vi "Main.vi"() -> ()   [LabVIEW 2020]
uses:
  Library Builder/Library Builder.lvclass
  Package Builder/Package Builder.lvclass
panel:
  in  "Stop":bool
  out "Time Elapsed":dbl format="%<%H:%M:%S>t"
  out "Status":string
  out "error out":errorcluster
  in  "Package Description":string="The NI-XNET Monitor Custom Device allows a user to run subordinate XNET session for each port in the system to be able to monitor port status, error counters, frame counter and other interface health indicators. This custom device also allows estimating the bus load present for the CAN buses added to the system. It's implemented as HW Inline Asynchronous Custom Device."
  in  "Build Config":T1(array[cluster])=[{"Version"=2020, "TCP/IP Port"=3363, "BuildPkg"=TRUE}, {"Version"=2021, "TCP/IP Port"=3364, "BuildPkg"=TRUE}, {"Version"=2023, "TCP/IP Port"=3365, "BuildPkg"=TRUE}]
  in  "Output Directory":path=path "\\\\vmware-host\\Shared Folders/_Repo/NI-XNET-Monitor-Custom-Device/Release"
  in  "Project Path":path=path "\\\\vmware-host\\Shared Folders/_Repo/NI-XNET-Monitor-Custom-Device/Source/NI-XNET Monitor Custom Device.lvproj"
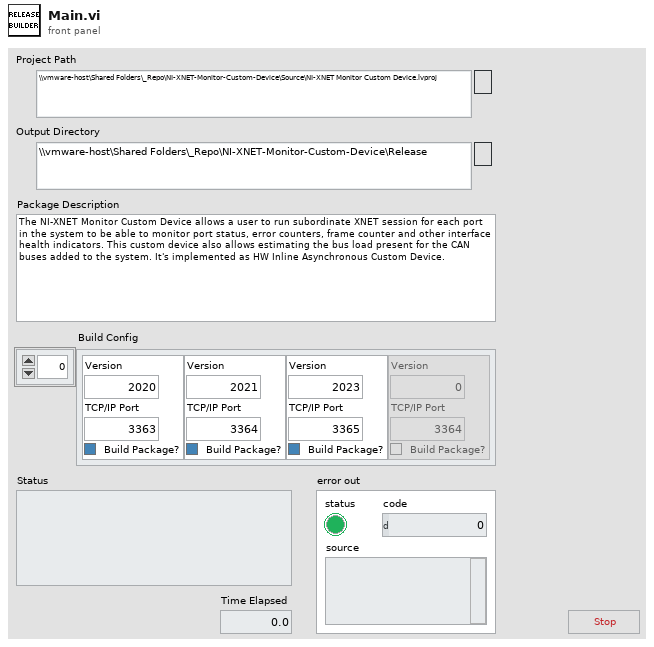
[diagram p1: front panel]
types:
  T1 = cluster{"Version":u32, "TCP/IP Port":i32, "BuildPkg":bool}[]
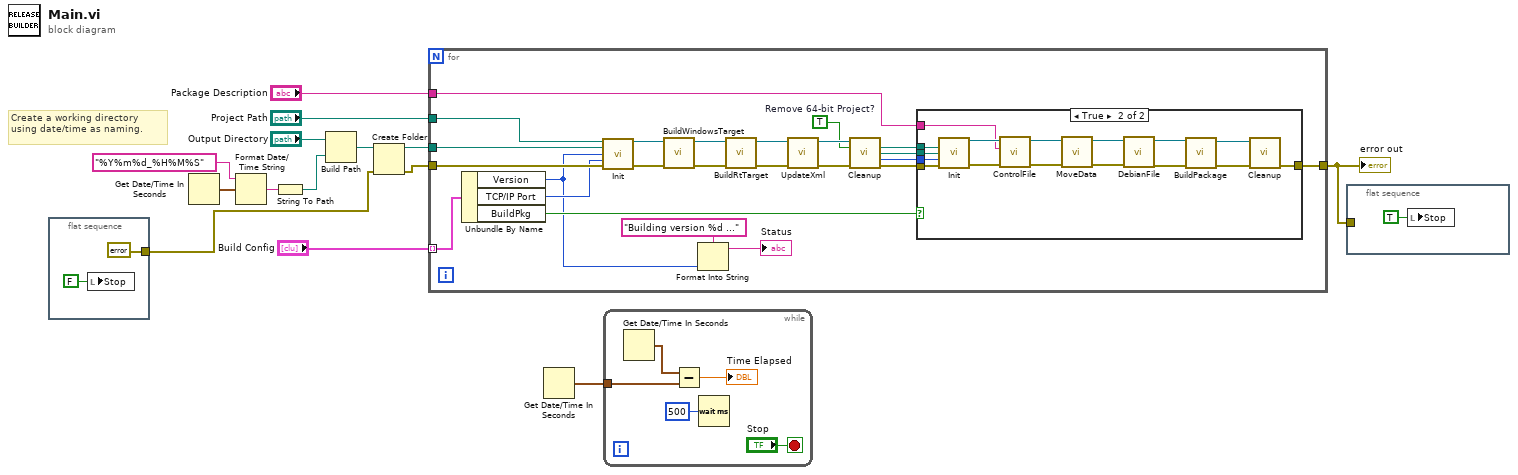
[diagram p0: block diagram]
diagram:
  # "Create a working directory using date/time as naming."
  n1 = flat-sequence {
    tunnel: [errorcluster {"status"=FALSE, "code"=0, "source"=""} ("error constant")] -> w2
    frame #0 {
      n2 = local write "Stop"(FALSE ("Stop")) -> ()
    }
  }
  n3 = Get Date/Time In Seconds() -> (seconds since 1Jan1904=w9:timestamp)
  n4 = Format Date/Time String(time format string (%c)="%Y%m%d_%H%M%S", seconds (now)=w9) -> (date/time string=w11:string)  [unwired: 1 in]
  n5 = String To Path(string=w11) -> (path=w12:path)
  n6 = Build Path(base path="Output Directory", name or relative path=w12) -> (appended path=w13:path)
  n7 = Create Folder(path (use dialog)=w13, error in=w2) -> (created path=w7:path, error out=w6:errorcluster)  [unwired: 1 in, 1 out]
  n8 = for {
    tunnel: "Project Path" -> [w40]
    tunnel: w7 -> [w35]
    tunnel: "Package Description" -> [w29]
    tunnel: "Build Config" -> [w22] mode=indexing
    tunnel: w6 -> [w34]
    tunnel: [w28] -> w1
    w23 = TRUE  # Remove 64-bit Project?
    n9 = Unbundle By Name(w22) -> ("Version"=w17:u32, "TCP/IP Port"=w21:i32, "BuildPkg"=w20:bool)
    n10 = call "Init.vi"("Project Path"=w40, "Working Directory"=w35, "Version"=w17, "TCP/IP Port"=w21, "error in (no error)"=w34) -> ("Library Builder out"=w39:refnum<class "Library Builder.lvclass">, "error out"=w38:errorcluster)  [unwired: 9 in]
    n11 = call "BuildWindowsTarget.vi"("error in (no error)"=w38, "Library Builder in"=w39) -> ("error out"=w36:errorcluster, "Library Builder out"=w37:refnum<class "Library Builder.lvclass">)  [unwired: 8 in]
    n12 = Format Into String(format string="Building version %d ...", w17) -> (resulting string=→"Status":string)  [unwired: 2 in, 1 out]
    n13 = call "BuildRtTarget.vi"("error in (no error)"=w36, "Library Builder in"=w37) -> ("error out"=w26:errorcluster, "Library Builder out"=w27:refnum<class "Library Builder.lvclass">)  [unwired: 8 in]
    n14 = call "UpdateXml.vi"("error in (no error)"=w26, "Library Builder in"=w27) -> ("error out"=w24:errorcluster, "Library Builder out"=w25:refnum<class "Library Builder.lvclass">)  [unwired: 8 in]
    n15 = call "Cleanup.vi"("Library Builder in"=w25, "Remove 64-bit Project?"=w23, "error in (no error)"=w24) -> ("Project Path"=w32:path, "Working Directory"=w31:path, "Version"=w30:u32, "error out"=w33:errorcluster)  [unwired: 8 in, 1 out]
    n16 = case shown="True" w20 {
      tunnel: w33 -> [w41 w57]
      tunnel: w32 -> [_ w56]
      tunnel: w31 -> [_ w55]
      tunnel: w30 -> [_ w54]
      tunnel: w29 -> [_ w52]
      tunnel: [w41 w42] -> w28
      frame False {
      }
      frame True {
        n17 = call "Init.vi"("Project Path"=w56, "Working Directory"=w55, "Version"=w54, "error in (no error)"=w57) -> ("Package Builder out"=w53:refnum<class "Package Builder.lvclass">, "error out"=w51:errorcluster)  [unwired: 10 in]
        n18 = call "ControlFile.vi"("error in (no error)"=w51, "Description"=w52, "Package Builder in"=w53) -> ("error out"=w49:errorcluster, "Package Builder out"=w50:refnum<class "Package Builder.lvclass">)  [unwired: 7 in]
        n19 = call "MoveData.vi"("error in (no error)"=w49, "Package Builder in"=w50) -> ("error out"=w47:errorcluster, "Package Builder out"=w48:refnum<class "Package Builder.lvclass">)  [unwired: 8 in]
        n20 = call "DebianFile.vi"("error in (no error)"=w47, "Package Builder in"=w48) -> ("error out"=w45:errorcluster, "Package Builder out"=w46:refnum<class "Package Builder.lvclass">)  [unwired: 8 in]
        n21 = call "BuildPackage.vi"("error in (no error)"=w45, "Package Builder in"=w46) -> ("error out"=w43:errorcluster, "Package Builder out"=w44:refnum<class "Package Builder.lvclass">)  [unwired: 8 in]
        n22 = call "Cleanup.vi"("error in (no error)"=w43, "Package Builder in"=w44) -> ("error out"=w42:errorcluster)  [unwired: 8 in, 1 out]
      }
    }
  }
  "error out" <- w1
  n23 = Get Date/Time In Seconds() -> (seconds since 1Jan1904=w3:timestamp)
  n24 = while {
    tunnel: w3 -> [w61]
    stop <- "Stop" stop-if-true
    n25 = Get Date/Time In Seconds() -> (seconds since 1Jan1904=w62:timestamp)
    n26 = Subtract(x=w62, y=w61) -> (x-y=→"Time Elapsed":dbl)
    n27 = Wait (ms)(milliseconds to wait=u32 500) -> ()  [unwired: 1 out]
  }
  n28 = flat-sequence {
    tunnel: w1 -> [_]
    frame #0 {
      n29 = local write "Stop"(TRUE ("Stop")) -> ()
    }
  }
